vi "emi_VI FP Background.vi"(0 "VI Refnum(This VI)":refnum<vi>, 1 "Width(Screen)":i32=-1, 2 "Height(Screen)":i32=-1, 3 "Dark(Black)":u32(colorbox), 4 "Light(White)":u32(colorbox)=16448250, 5 "error in":errorcluster, 6 "Graphic Type(Flat Color)":T1, 7 "Pane Index (-1=all)":i32=-1) -> (14 "VI Refnum out":refnum<vi>, 19 "error IO":errorcluster)   [LabVIEW 2011]
doc: "Set the background graphic for a VIs frontpanel. \nNote that With and height must be bigger then the largest size for the FP. If left blank, a background the size of the screen is generated.\n\nIn pane index, the index of the pane to use may be input. If it is omited, all panes will be changed.\n\nOn error: No action performed"
uses:
  0 - General/Graphix/Private/emi_List Of Graphix.ctl
  <vilib>/picture/picture.llb/imagedata.ctl
  0 - General/Graphix/emi_BW 8Bit image to Linear DuoTone.vi
  0 - General/Graphix/emi_Tile Gradient Image.vi
  <vilib>/picture/picture.llb/Draw Flattened Pixmap.vi
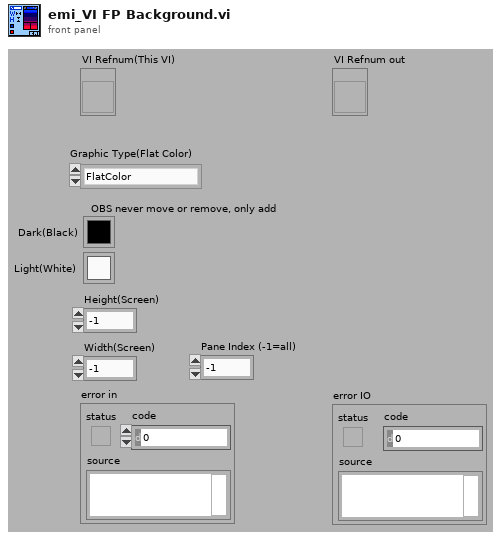
[diagram p1: front panel]
types:
  T1 = typedef "emi_List Of Graphix.ctl" = enum16{"FlatColor", "SharpGrad", "ShallowGrad", "GlasGradBord", "GlasGrad", "GlasGradBord 2"}
  T2 = typedef "imagedata.ctl" = cluster{"image type":i32, "image depth":i32, "image":u8[], "mask":u8[], "colors":u32[], "Rectangle":cluster{"left":i16, "top":i16, "right":i16, "bottom":i16}}
  T3 = typedef "LVRectTypeDef.ctl" = cluster{"left":i16, "top":i16, "right":i16, "bottom":i16}
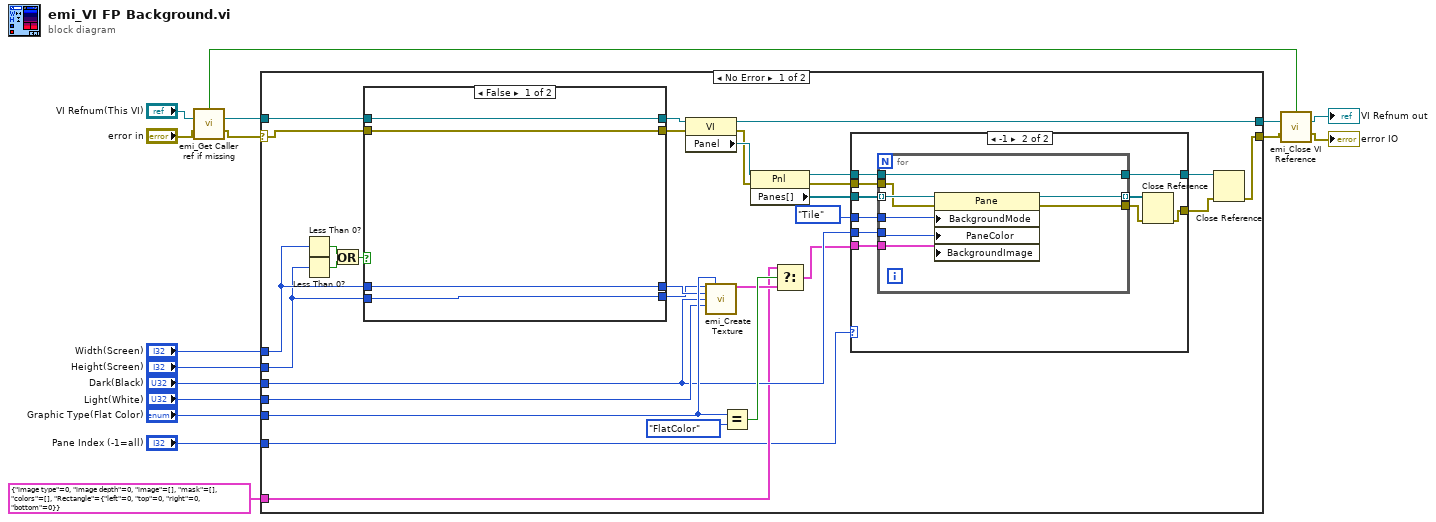
[diagram p0: block diagram]
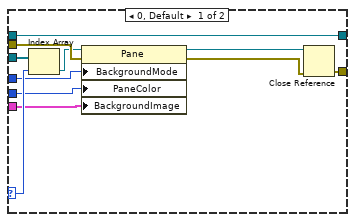
[diagram p2: hidden frame]
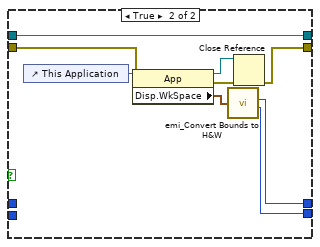
[diagram p3: hidden frame]
diagram:
  n1 = call "emi_Get Caller ref if missing.vi"("VI Refnum(Calling VI)"="VI Refnum(This VI)", "error in (no error)"="error in") -> ("Ref Generated"=w10:bool, "VI Refnum Out"=w1:refnum<vi>, "error out"=w4:errorcluster)  [unwired: 11 in]
  n2 = case shown="No Error" w4 {
    selector: w4 -> [w37 w90]
    tunnel: "Graphic Type(Flat Color)" -> [w45 _]
    tunnel: T2 {"image type"=0, "image depth"=0, "image"=[], "mask"=[], "colors"=[], "Rectangle"={"left"=0, "top"=0, "right"=0, "bottom"=0}} ("Image Data Out") -> [w26 _]
    tunnel: "Width(Screen)" -> [w40 _]
    tunnel: "Height(Screen)" -> [w39 _]
    tunnel: "Dark(Black)" -> [w28 _]
    tunnel: "Light(White)" -> [w44 _]
    tunnel: [w20 w90] -> w6
    tunnel: [w21 w89] -> w8
    tunnel: "Pane Index (-1=all)" -> [w19 _]
    tunnel: w1 -> [w17 w89]
    frame No Error {
      n3 = Less Than 0?(x=w40) -> (x < 0?=w41:bool)
      n4 = Less Than 0?(x=w39) -> (x < 0?=w42:bool)
      n5 = Or(x=w41, y=w42) -> (x .or. y?=w38:bool)
      n6 = case shown="False" w38 {
        tunnel: w37 -> [w79 w87]
        tunnel: [w79 w81] -> w32
        tunnel: w40 -> [w78 _]
        tunnel: [w78 w85] -> w36
        tunnel: w39 -> [w77 _]
        tunnel: [w77 w84] -> w35
        tunnel: [w76 w80] -> w18
        tunnel: w17 -> [w76 w80]
        frame False {
        }
        frame True {
          n7 = control-ref of="This Application"() -> (w88:refnum<vi>)
          n8 = property class="App"(reference=w88, error in=w87) -> (reference out=w82:refnum<vi>, error out=w83:errorcluster, "Disp.WkSpace"=w86:T3)
          n9 = call "emi_Convert Bounds to H&W.vi"("Bounds"=w86) -> ("Width"=w85:i32, "Height"=w84:i32)  [unwired: 6 in]
          n10 = Close Reference(reference=w82, error in (no error)=w83) -> (error out=w81:errorcluster)
        }
      }
      n11 = property class="VI"(reference=w18, error in=w32) -> (reference out=w21:refnum<vi>, error out=w33:errorcluster, "Panel"=w34:refnum<vi>)
      n12 = call "emi_Create Texture.vi"("Height(600)"=w35, "Graphic Type(Flat Color)"=w45, "Width(400)"=w36, "Dark(Black)"=w28, "Light(White)"=w44) -> ("Image Data Out"=w27:T2)  [unwired: 8 in, 2 out]
      n13 = Equal?(x=w45, y=emi_List_Of_Graphix."FlatColor" ("Graphic Type")) -> (x = y?=w43:bool)
      n14 = property class="Pnl"(reference=w34, error in=w33) -> (reference out=w24:refnum<vi>, error out=w30:errorcluster, "Panes[]"=w31:refnum<vi>[])
      n15 = Select(t=w26, s=w43, f=w27) -> (s? t:f=w25:T2)
      n16 = case shown="-1" w19 {
        selector: w19 -> [w56 _]
        tunnel: w31 -> [w57 w67]
        tunnel: w30 -> [w51 w66]
        tunnel: enum16{"Stretch", "Center", "Tile"}."Tile" ("Background Mode") -> [w49 w65]
        tunnel: w28 -> [w48 w64]
        tunnel: w25 -> [w47 w63]
        tunnel: w24 -> [w54 w60]
        tunnel: [w55 w59] -> w23
        tunnel: [w54 w58] -> w22
        frame 0, Default {
          n17 = Index Array(array=w57, index=w56) -> (element=w50:refnum<vi>)
          n18 = property class="Pane"(reference=w50, error in=w51, "BackgroundMode"=w49, "PaneColor"=w48, "BackgroundImage"=w47) -> (reference out=w53:refnum<vi>, error out=w52:errorcluster)
          n19 = Close Reference(reference=w53, error in (no error)=w52) -> (error out=w55:errorcluster)
        }
        frame -1 {
          n20 = for {
            tunnel: w67 -> [w75] mode=indexing
            tunnel: w66 -> [w74]
            tunnel: w65 -> [w73]
            tunnel: w64 -> [w72]
            tunnel: w63 -> [w71]
            tunnel: [w70] -> w61 mode=indexing
            tunnel: [w69] -> w62
            tunnel: w60 -> [w68]
            tunnel: [w68] -> w58
            n21 = property class="Pane"(reference=w75, error in=w74, "BackgroundMode"=w73, "PaneColor"=w72, "BackgroundImage"=w71) -> (reference out=w70:refnum<vi>, error out=w69:errorcluster)
          }
          n22 = Close Reference(reference=w61, error in (no error)=w62) -> (error out=w59:errorcluster)
        }
      }
      n23 = Close Reference(reference=w22, error in (no error)=w23) -> (error out=w20:errorcluster)
    }
    frame Error {
    }
  }
  n24 = call "emi_Close VI Reference.vi"("Close ref?(T)"=w10, "VI Refnum"=w8, "error in (no error)"=w6) -> ("VI Refnum Out"=→"VI Refnum out":refnum<vi>, "error out"=→"error IO":errorcluster)  [unwired: 11 in]
